vi "ElevadorLabView.vi"() -> ()   [LabVIEW 2012]
uses:
  <vilib>/Instr/_visa.llb/VISA Configure Serial Port (Instr).vi
panel:
  in  "EMERGENCIA VERIFICADA":bool
  out "Emergencia":bool
  out "Erro Fim de Curso":bool
  in  "EMERGENCIA":bool
  in  "INT 4":bool
  in  "INT 3":bool
  in  "INT 2":bool
  in  "INT 1":bool
  out "Comunicou":bool
  out "Andar Atual":dbl
  out "FC 1":bool
  out "FC 2":bool
  out "FC 3":bool
  out "FC 4":bool
  out "read buffer":string
  out "Ext Desc 2":bool
  out "Ext 1":bool
  out "Ext 4":bool
  out "Ext Sobe 3":bool
  out "Ext Desc 3":bool
  out "Ext Sobe 2":bool
  out "Int 1":bool
  out "Int 2":bool
  out "Int 3":bool
  out "Int 4":bool
  in  "Turn On":bool
  in  "Stop Button":bool
  in  "Baud Rate":u32=9600
  in  "COM Port":refnum<visa-resource-name>
  out "Available?":bool
  # "Começa a Comunicação"
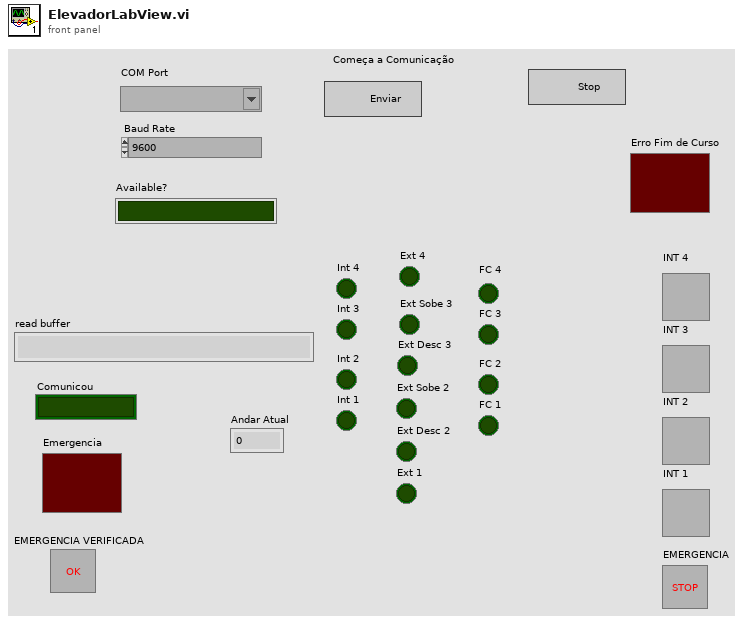
[diagram p1: front panel]
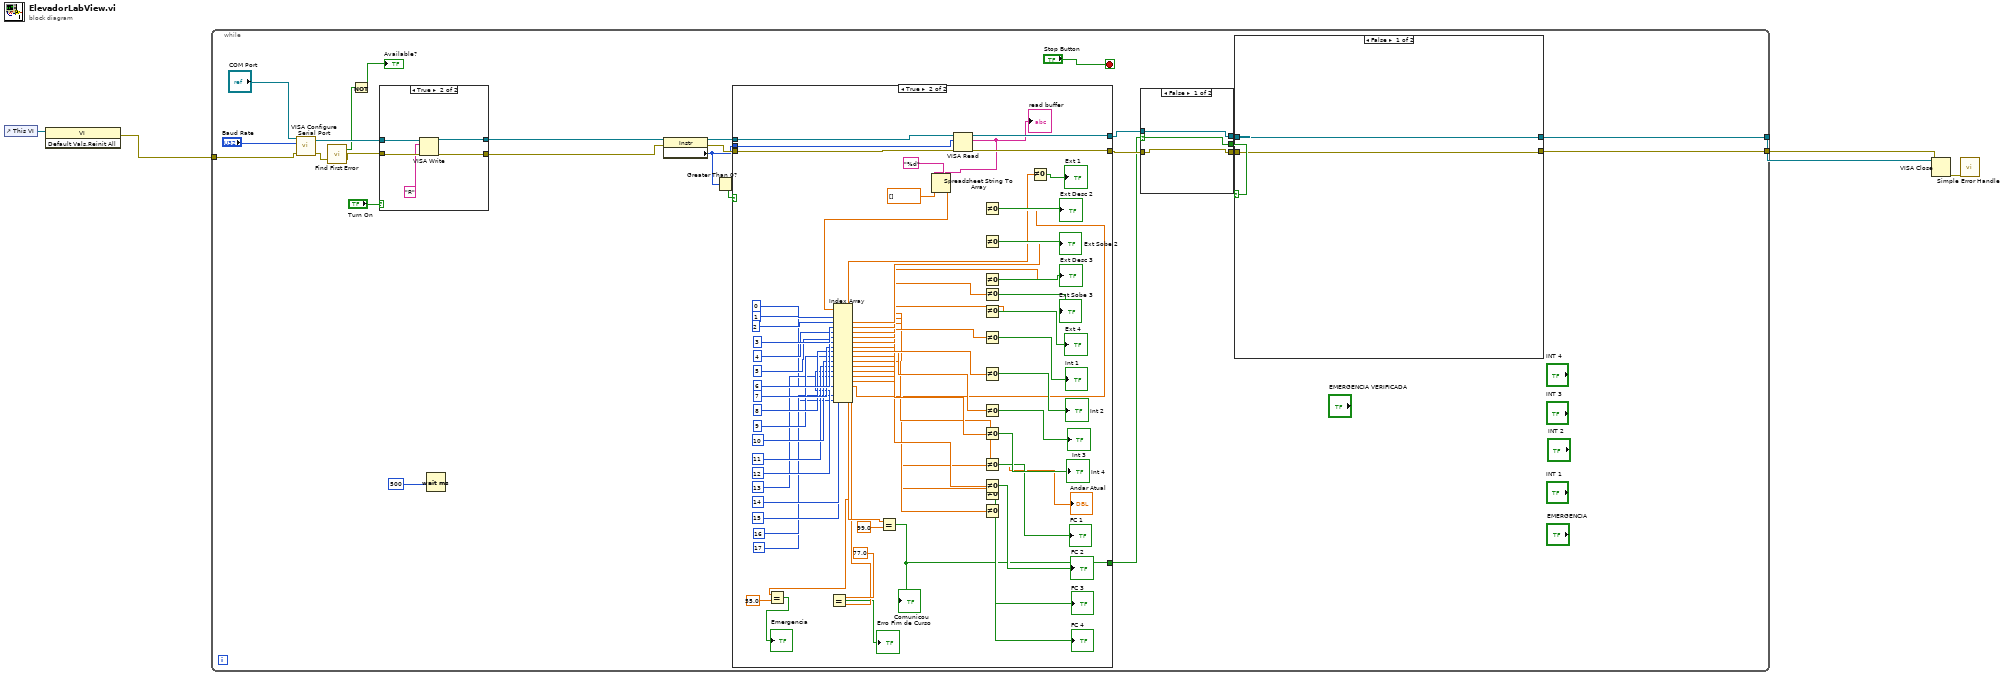
[diagram p0: block diagram]
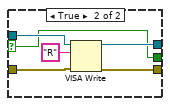
[diagram p2: hidden frame]
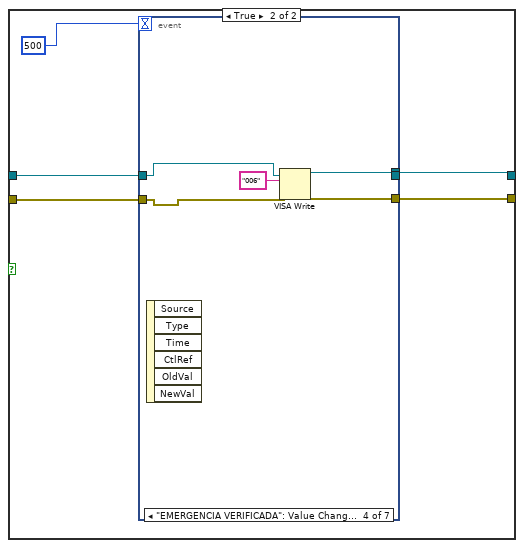
[diagram p3: hidden frame]
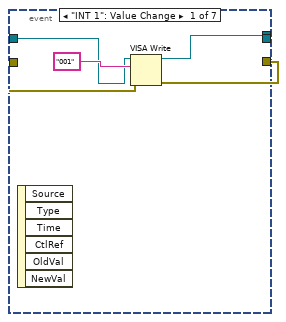
[diagram p4: hidden frame]
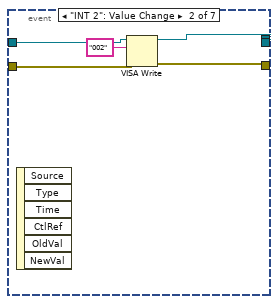
[diagram p5: hidden frame]
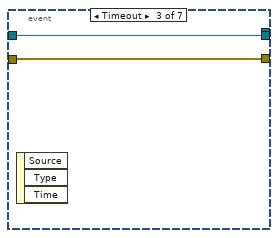
[diagram p6: hidden frame]
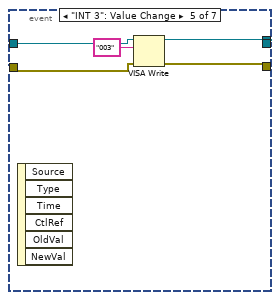
[diagram p7: hidden frame]
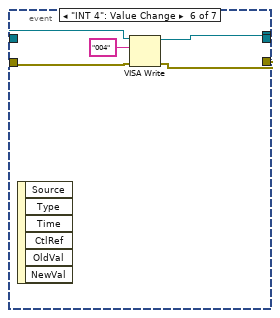
[diagram p8: hidden frame]
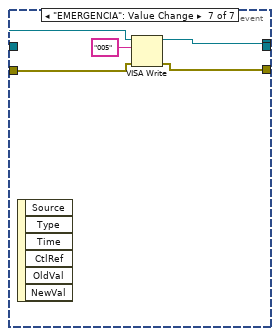
[diagram p9: hidden frame]
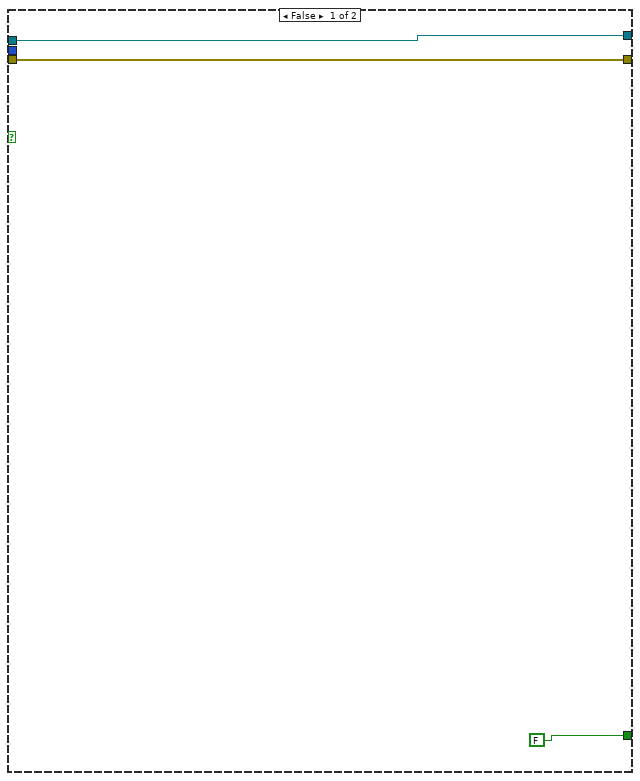
[diagram p10: hidden frame]
diagram:
  n1 = control-ref of="This VI"() -> (w1:refnum<vi>)
  n2 = invoke class="VI" method="Default Vals.Reinit All"(reference=w1) -> (error out=w2:errorcluster)  [unwired: 2 in, 2 out]
  n3 = while {
    tunnel: [w13] -> w4
    tunnel: [w14] -> w5
    tunnel: w2 -> [w18]
    stop <- "Stop Button" stop-if-true
    n4 = call-poly "VISA Configure Serial Port"("VISA resource name"="COM Port", "baud rate (9600)"="Baud Rate", "error in (no error)"=w18) -> ("VISA resource name out"=w23:refnum<visa-resource-name>, "error out"=w21:errorcluster)  [unwired: 11 in]
    n5 = call <vilib>:"Find First Error.vi"("error in (no error)"=w21) -> ("error out"=w22:errorcluster, "error?"=w20:bool)  [unwired: 3 in]
    n6 = Not(x=w20) -> (.not. x?=→"Available?":bool)
    n7 = case shown="True" "Turn On" {
      tunnel: [w148 w153] -> w16
      tunnel: [w147 w152] -> w15
      tunnel: w23 -> [w148 w151]
      tunnel: w22 -> [w147 w150]
      frame False {
      }
      frame True {
        n8 = VISA Write(VISA resource name=w151, write buffer="R", error in (no error)=w150) -> (VISA resource name out=w153:refnum<visa-resource-name>, error out=w152:errorcluster)  [unwired: 1 out]
      }
    }
    n9 = Wait (ms)(milliseconds to wait=u32 500 ("millisecond timer value")) -> ()  [unwired: 1 out]
    n10 = property class="Instr"(reference=w16, error in=w15) -> (reference out=w28:refnum<visa-resource-name>, error out=w29:errorcluster, "Serial Settings:Number of Bytes at Serial Port"=w17:u32)
    n11 = Greater Than 0?(x=w17) -> (x > 0?=w30:bool)
    n12 = case shown="True" w30 {
      tunnel: w28 -> [w81 w130]
      tunnel: w29 -> [w80 w129]
      tunnel: [w81 w146] -> w11
      tunnel: [w80 w145] -> w10
      tunnel: w17 -> [_ w128]
      tunnel: [FALSE w91] -> w7
      frame False {
      }
      frame True {
        n13 = VISA Read(VISA resource name=w130, byte count=w128, error in (no error)=w129) -> (VISA resource name out=w146:refnum<visa-resource-name>, read buffer=w126:string, error out=w145:errorcluster)  [unwired: 1 out]
        "read buffer" <- w126
        n14 = Spreadsheet String To Array(format string="%d", spreadsheet string=w126, array type (2D Dbl)=dbl[] []) -> (array=w90:dbl[])  [unwired: 1 in]
        n15 = Index Array(array=w90, index #1=0 ("index"), index #2=2 ("index"), index #3=3 ("index"), index #4=4 ("index"), index #5=5 ("index"), index #6=6 ("index"), index #7=7 ("index"), index #8=8 ("index"), index #9=9 ("index"), index #10=10 ("index"), index #11=11 ("index"), index #12=12 ("index"), index #13=13 ("index"), index #14=14 ("index"), index #15=1 ("index"), index #16=15 ("index"), index #17=16 ("index"), index #18=17 ("index")) -> (element #1=w124:dbl, element #2=w123:dbl, element #3=w122:dbl, element #4=w121:dbl, element #5=w120:dbl, element #6=w119:dbl, element #7=w118:dbl, element #8=w117:dbl, element #9=w116:dbl, element #10=w115:dbl, element #11=w114:dbl, element #12=w113:dbl, element #13=w112:dbl, element #14=→"Andar Atual":dbl, element #15=w96:dbl, element #16=w93:dbl, element #17=w87:dbl, element #18=w84:dbl)
        n16 = Equal?(x=w84, y=55.0) -> (x = y?=→"Emergencia":bool)
        n17 = Equal?(x=77.0 ("y"), y=w87) -> (x = y?=→"Erro Fim de Curso":bool)
        n18 = Equal?(x=w93, y=99.0) -> (x = y?=w91:bool)
        "Comunicou" <- w91
        n19 = Not Equal To 0?(x=w96) -> (x != 0?=→"Ext Desc 2":bool)
        n20 = Not Equal To 0?(x=w123) -> (x != 0?=→"Ext Sobe 2":bool)
        n21 = Not Equal To 0?(x=w122) -> (x != 0?=→"Ext Desc 3":bool)
        n22 = Not Equal To 0?(x=w121) -> (x != 0?=→"Ext Sobe 3":bool)
        n23 = Not Equal To 0?(x=w120) -> (x != 0?=→"Ext 4":bool)
        n24 = Not Equal To 0?(x=w119) -> (x != 0?=→"Int 1":bool)
        n25 = Not Equal To 0?(x=w118) -> (x != 0?=→"Int 2":bool)
        n26 = Not Equal To 0?(x=w117) -> (x != 0?=→"Int 3":bool)
        n27 = Not Equal To 0?(x=w116) -> (x != 0?=→"Int 4":bool)
        n28 = Not Equal To 0?(x=w115) -> (x != 0?=→"FC 1":bool)
        n29 = Not Equal To 0?(x=w114) -> (x != 0?=→"FC 2":bool)
        n30 = Not Equal To 0?(x=w112) -> (x != 0?=→"FC 4":bool)
        n31 = Not Equal To 0?(x=w113) -> (x != 0?=→"FC 3":bool)
        n32 = Not Equal To 0?(x=w124) -> (x != 0?=→"Ext 1":bool)
      }
    }
    n33 = case shown="False" w7 {
      selector: w7 -> [w31 w34]
      tunnel: w11 -> [w33 w38]
      tunnel: w10 -> [w32 w37]
      tunnel: [w32 w36] -> w9
      tunnel: [w33 w35] -> w8
      tunnel: [w31 w34] -> w6
      frame False {
      }
      frame True {
        n34 = VISA Write(VISA resource name=w38, write buffer="R", error in (no error)=w37) -> (VISA resource name out=w35:refnum<visa-resource-name>, error out=w36:errorcluster)  [unwired: 1 out]
      }
    }
    n35 = case shown="False" w6 {
      tunnel: w8 -> [w41 w46]
      tunnel: w9 -> [w40 w45]
      tunnel: [w40 w44] -> w14
      tunnel: [w41 w43] -> w13
      frame False {
      }
      frame True {
        n36 = event shown="[3] \"EMERGENCIA VERIFICADA\": Value Change" {
          selector: _ -> [_ _ _ _ _ _ _]
          dyn-events: _ -> [_ _ _ _ _ _ _]
          timeout: u32 500 ("milliseconds to wait") -> [_ _ _ _ _ _ _]
          tunnel: w46 -> [w50 w55 w58 w61 w67 w69 w74]
          tunnel: w45 -> [w49 w54 w57 w62 w66 w70 w75]
          tunnel: [w48 w53 w57 w59 w65 w71 w76] -> w44
          tunnel: [w47 w52 _ w60 w64 w72 w77] -> w43
          tunnel: [_ _ w58 _ _ _ _] -> _
          event "INT 1": Value Change {
            n37 = event-data() -> ()  [unwired: 1 in, 6 out]
            n38 = VISA Write(VISA resource name=w50, write buffer="001", error in (no error)=w49) -> (VISA resource name out=w47:refnum<visa-resource-name>, error out=w48:errorcluster)  [unwired: 1 out]
          }
          event "INT 2": Value Change {
            n39 = event-data() -> ()  [unwired: 1 in, 6 out]
            n40 = VISA Write(VISA resource name=w55, write buffer="002", error in (no error)=w54) -> (VISA resource name out=w52:refnum<visa-resource-name>, error out=w53:errorcluster)  [unwired: 1 out]
          }
          event Timeout {
            n41 = event-data() -> ()  [unwired: 1 in, 3 out]
          }
          event "EMERGENCIA VERIFICADA": Value Change {
            n42 = event-data() -> ()  [unwired: 1 in, 6 out]
            n43 = VISA Write(VISA resource name=w61, write buffer="006", error in (no error)=w62) -> (VISA resource name out=w60:refnum<visa-resource-name>, error out=w59:errorcluster)  [unwired: 1 out]
          }
          event "INT 3": Value Change {
            n44 = event-data() -> ()  [unwired: 1 in, 6 out]
            n45 = VISA Write(VISA resource name=w67, write buffer="003", error in (no error)=w66) -> (VISA resource name out=w64:refnum<visa-resource-name>, error out=w65:errorcluster)  [unwired: 1 out]
          }
          event "INT 4": Value Change {
            n46 = event-data() -> ()  [unwired: 1 in, 6 out]
            n47 = VISA Write(VISA resource name=w69, write buffer="004", error in (no error)=w70) -> (VISA resource name out=w72:refnum<visa-resource-name>, error out=w71:errorcluster)  [unwired: 1 out]
          }
          event "EMERGENCIA": Value Change {
            n48 = event-data() -> ()  [unwired: 1 in, 6 out]
            n49 = VISA Write(VISA resource name=w74, write buffer="005", error in (no error)=w75) -> (VISA resource name out=w77:refnum<visa-resource-name>, error out=w76:errorcluster)  [unwired: 1 out]
          }
        }
      }
    }
  }
  n50 = VISA Close(VISA resource name=w4, error in (no error)=w5) -> (error out=w3:errorcluster)
  n51 = call <vilib>:"Simple Error Handler.vi"("error in (no error)"=w3) -> ()  [unwired: 4 in, 5 out]
